vi "Page_Advanced_Initialize.vi"(6 "ctl references":T1, 8 "error in (no error)":errorcluster, 11 "AB_Build in":refnum<class "AB_Build.lvclass">) -> (0 "error out":errorcluster, 3 "AB_Build out":refnum<class "AB_Build.lvclass">)   [LabVIEW 2020, in "AB_Build.lvclass"]
uses:
  <vilib>/AppBuilder/AB_Classes/Build/AB_Build.lvclass
  <resource>/Framework/Providers/Builds/AppBuilder/AB_UI_Page_Advanced_References.ctl
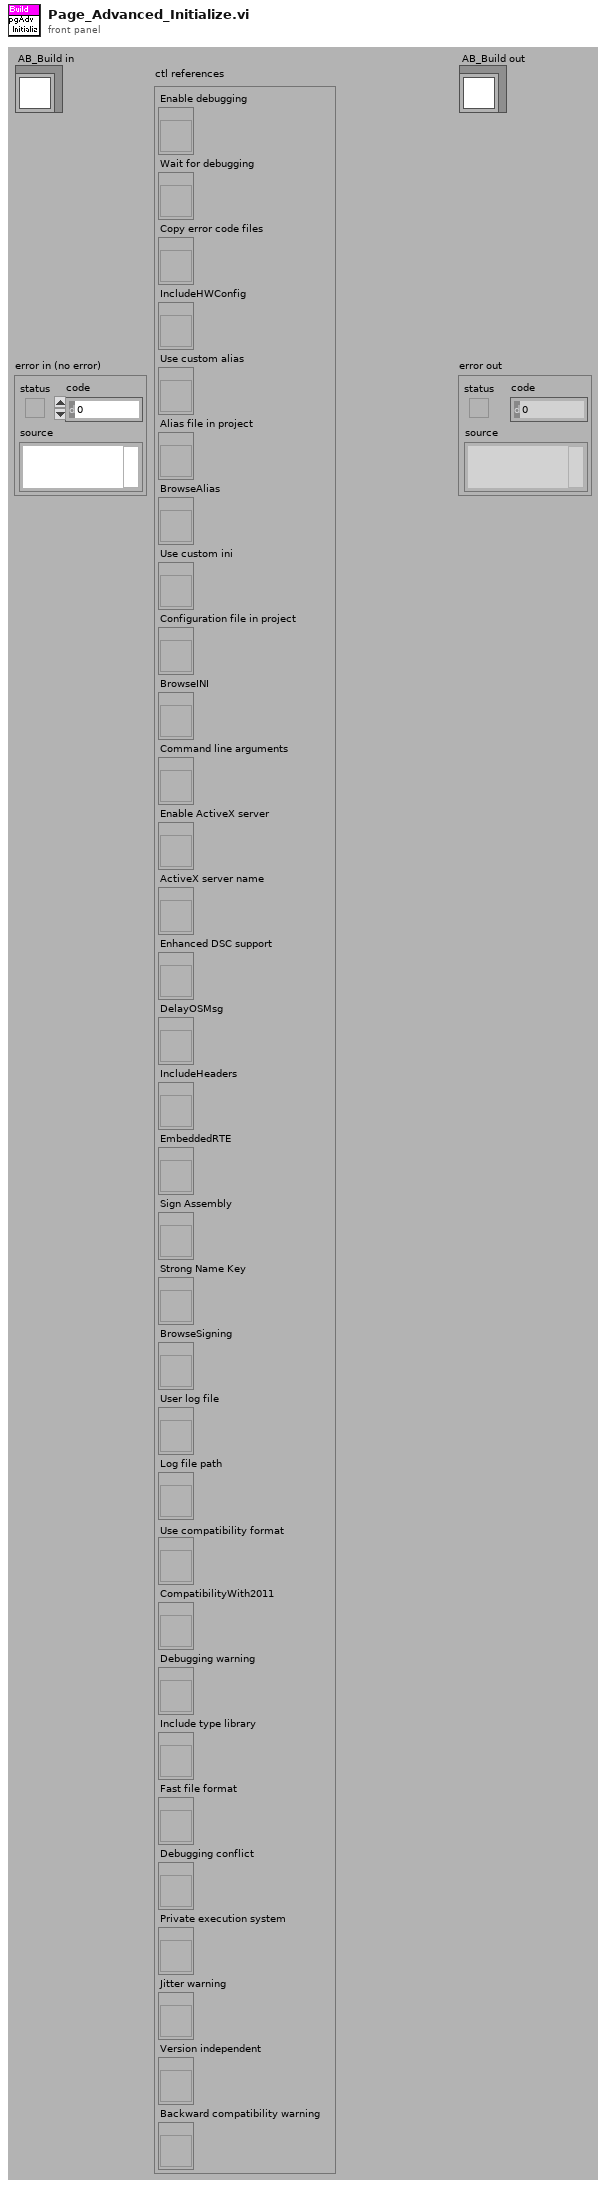
[diagram p1: front panel]
types:
  T1 = typedef "AB_UI_Page_Advanced_References.ctl" = cluster{"Enable debugging":refnum<vi>, "Wait for debugging":refnum<vi>, "Copy error code files":refnum<vi>, "IncludeHWConfig":refnum<vi>, "Use custom alias":refnum<vi>, "Alias file in project":refnum<vi>, "BrowseAlias":refnum<vi>, "Use custom ini":refnum<vi>, "Configuration file in project":refnum<vi>, "BrowseINI":refnum<vi>, "Command line arguments":refnum<vi>, "Enable ActiveX server":refnum<vi>, "ActiveX server name":refnum<vi>, "Enhanced DSC support":refnum<vi>, "DelayOSMsg":refnum<vi>, "IncludeHeaders":refnum<vi>, "EmbeddedRTE":refnum<vi>, "Sign Assembly":refnum<vi>, "Strong Name Key":refnum<vi>, "BrowseSigning":refnum<vi>, "User log file":refnum<vi>, "Log file path":refnum<vi>, "Use compatibility format":refnum<vi>, "CompatibilityWith2011":refnum<vi>, "Debugging warning":refnum<vi>, "Include type library":refnum<vi>, "Fast file format":refnum<vi>, "Debugging conflict":refnum<vi>, "Private execution system":refnum<vi>, "Jitter warning":refnum<vi>, "Version independent":refnum<vi>, "Backward compatibility warning":refnum<vi>}
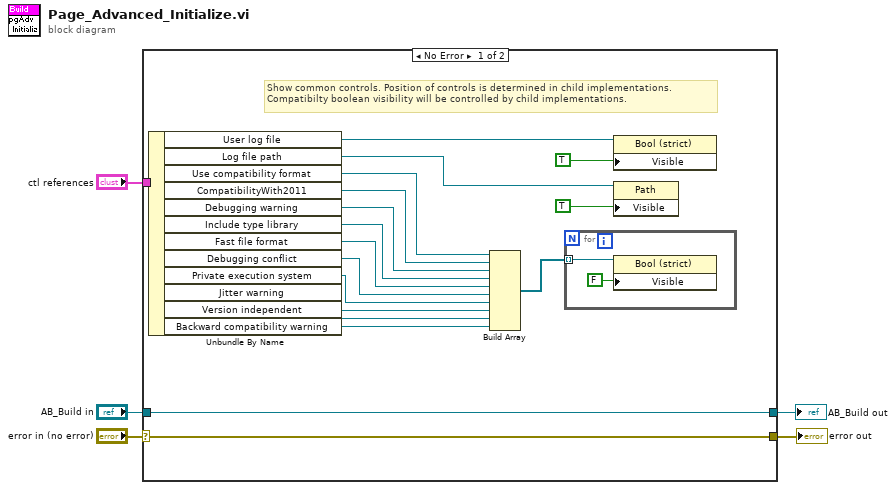
[diagram p0: block diagram]
diagram:
  n1 = case shown="No Error" "error in (no error)" {
    selector: "error in (no error)" -> [w17 w27]
    tunnel: [w17 w27] -> w4
    tunnel: [w18 w26] -> w2
    tunnel: "AB_Build in" -> [w18 w26]
    tunnel: "ctl references" -> [w23 _]
    frame No Error {
      # "Show common controls. Position of controls is determined in child implementations.\nCompatibilty boolean visibility will be controlled by child implementations."
      n2 = Unbundle By Name(w23) -> ("User log file"=w22:refnum<vi>, "Log file path"=w21:refnum<vi>, "Use compatibility format"=w14:refnum<vi>, "CompatibilityWith2011"=w16:refnum<vi>, "Debugging warning"=w15:refnum<vi>, "Include type library"=w12:refnum<vi>, "Fast file format"=w11:refnum<vi>, "Debugging conflict"=w10:refnum<vi>, "Private execution system"=w9:refnum<vi>, "Jitter warning"=w8:refnum<vi>, "Version independent"=w7:refnum<vi>, "Backward compatibility warning"=w6:refnum<vi>)
      n3 = Build Array(w14, w16, w15, w12, w11, w10, w9, w8, w7, w6) -> (w13:refnum<vi>[])
      n4 = for {
        tunnel: w13 -> [w24] mode=indexing
        n5 = property class="Bool (strict)"(reference=w24, "Visible"=FALSE) -> ()  [unwired: 1 in, 2 out]
      }
      n6 = property class="Bool (strict)"(reference=w22, "Visible"=TRUE) -> ()  [unwired: 1 in, 2 out]
      n7 = property class="Path"(reference=w21, "Visible"=TRUE) -> ()  [unwired: 1 in, 2 out]
    }
    frame Error {
    }
  }
  "error out" <- w4
  "AB_Build out" <- w2
